vi "Progress Bar - Manager.vi"(6 "Steps to Increment (1)":dbl=1.0, 7 "Action (Init)":T1, 8 "error in (no error)":errorcluster, 9 "Number of Steps":dbl, 10 "Window Title (\"\")":string, 11 "Message":string) -> (0 "error out":errorcluster)   [LabVIEW 2014, in "Progress Bar.lvlib"]
uses:
  Progress Bar.lvlib
  _typedefs/PB_Manager Actions.ctl
  _typedefs/PB_Ref Cluster.ctl
panel:
  out "Init - Timed Out":bool
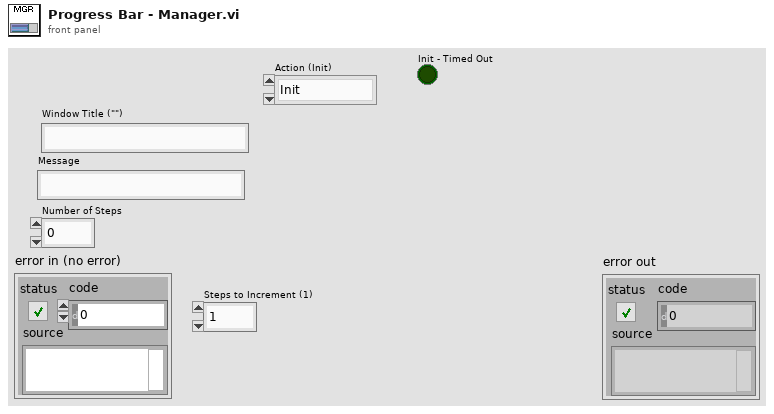
[diagram p1: front panel]
types:
  T1 = typedef "PB_Manager Actions.ctl" = enum16{"Init", "Update Bar", "Close"}
  T2 = typedef "PB_Ref Cluster.ctl" = cluster{"Message":refnum<user-event>, "ShutDown":refnum<user-event>, "User Abort":refnum<notifier>, "Load Complete":refnum<notifier>}
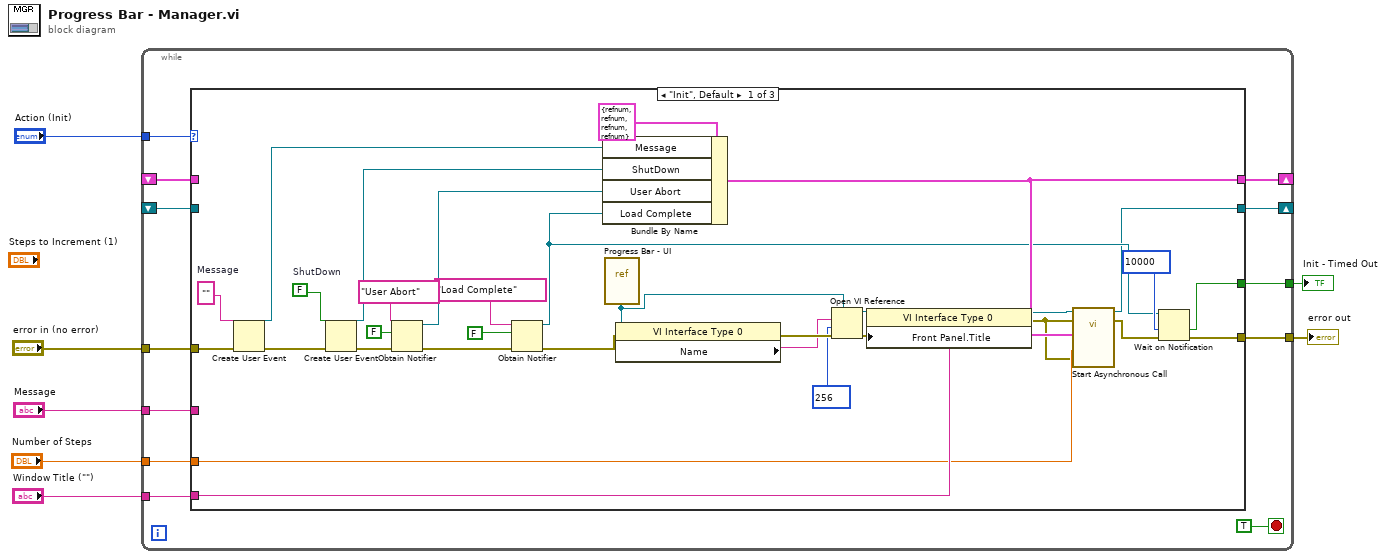
[diagram p0: block diagram]
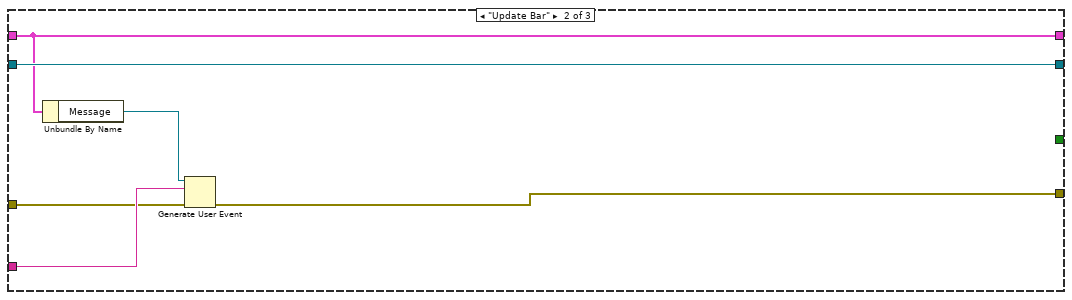
[diagram p2: hidden frame]
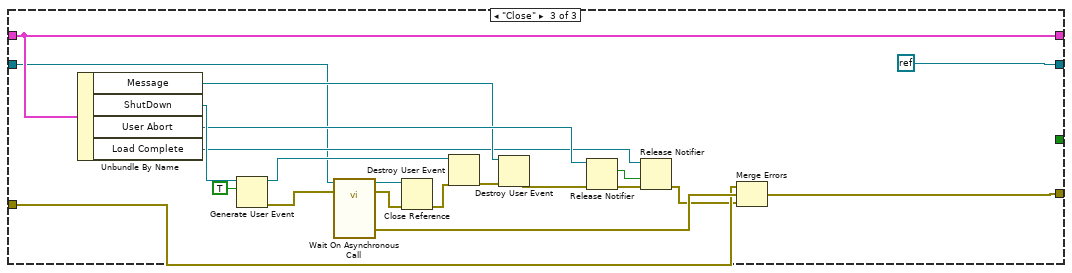
[diagram p3: hidden frame]
diagram:
  n1 = while {
    tunnel: "Action (Init)" -> [w19]
    shift-right: [w17] -> _
    shift-left: _ -> [w12]
    tunnel: "error in (no error)" -> [w16]
    tunnel: "Number of Steps" -> [w15]
    tunnel: [w14] -> w4
    shift-right: [w13] -> _
    shift-left: _ -> [w11]
    tunnel: "Message" -> [w10]
    tunnel: "Window Title (\"\")" -> [w9]
    tunnel: [w8] -> w1
    stop <- TRUE stop-if-true
    n2 = case shown="\"Init\", Default" w19 {
      tunnel: [w40 w52 w65] -> w17
      tunnel: w16 -> [w50 w54 w63]
      tunnel: w15 -> [w21 _ _]
      tunnel: [w29 w53 w66] -> w14
      tunnel: [w22 w57 refnum<k0> refnum] -> w13
      tunnel: w12 -> [_ w52 w65]
      tunnel: w11 -> [_ w57 w58]
      tunnel: w10 -> [_ w55 _]
      tunnel: w9 -> [w24 _ _]
      tunnel: [w28 _ _] -> w8
      frame "Init", Default {
        w48 = FALSE  # ShutDown
        w49 = ""  # Message
        n3 = Create User Event(user event datatype=w49, error in=w50) -> (user event=w41:refnum<user-event>, error out=w47:errorcluster)
        n4 = Create User Event(user event datatype=w48, error in=w47) -> (user event=w42:refnum<user-event>, error out=w45:errorcluster)
        n5 = Obtain Notifier(name (unnamed)="User Abort", notification data type=FALSE, error in (no error)=w45) -> (notifier out=w44:refnum<notifier>, error out=w33:errorcluster)  [unwired: 1 in, 1 out]
        n6 = Obtain Notifier(name (unnamed)="Load Complete", notification data type=FALSE, error in (no error)=w33) -> (notifier out=w30:refnum<notifier>, error out=w32:errorcluster)  [unwired: 1 in, 1 out]
        n7 = Bundle By Name(cluster=T2 {"Message"=refnum, "ShutDown"=refnum, "User Abort"=refnum, "Load Complete"=refnum} ("PB_Ref Cluster"), "Message"=w41, "ShutDown"=w42, "User Abort"=w44, "Load Complete"=w30) -> (w40:T2)
        n8 = vi-ref "Progress Bar - UI.vi"() -> (w37:refnum<vi>)
        n9 = property class="VI Interface Type 0"(reference=w37, error in=w32) -> (error out=w39:errorcluster, "Name"=w38:string)  [unwired: 1 out]
        n10 = Open VI Reference(type specifier VI Refnum (for type only)=w37, vi path=w38, options=256, error in (no error)=w39) -> (vi reference=w26:refnum<vi>, error out=w25:errorcluster)  [unwired: 2 in]
        n11 = property class="VI Interface Type 0"(reference=w26, error in=w25, "Front Panel.Title"=w24) -> (reference out=w23:refnum<vi>, error out=w20:errorcluster)
        n12 = call-by-ref "Start Asynchronous Call"(reference=w23, error in=w20, 8:"error in (no error)"=w20, "Number of Steps"=w21, "Ref Cluster"=w40) -> (reference out=w22:refnum<vi>, error out=w27:errorcluster)  [unwired: 8 in, 1 out]
        n13 = Wait on Notification(notifier=w30, timeout in ms (-1)=10000, error in (no error)=w27) -> (timed out?=w28:bool, error out=w29:errorcluster)  [unwired: 1 in, 2 out]
      }
      frame "Update Bar" {
        n14 = Unbundle By Name(w52) -> ("Message"=w56:refnum<user-event>)
        n15 = Generate User Event(user event=w56, event data cluster=w55, error in=w54) -> (error out=w53:errorcluster)  [unwired: 1 in, 1 out]
      }
      frame "Close" {
        n16 = Unbundle By Name(w65) -> ("Message"=w71:refnum<user-event>, "ShutDown"=w78:refnum<user-event>, "User Abort"=w72:refnum<notifier>, "Load Complete"=w60:refnum<notifier>)
        n17 = Generate User Event(user event=w78, event data cluster=TRUE ("event data")) -> (user event out=w73:refnum<user-event>, error out=w76:errorcluster)  [unwired: 2 in]
        n18 = call-by-ref "Wait On Asynchronous Call"(reference=w58, error in=w76) -> (reference out=w69:refnum<vi>, error out=w68:errorcluster, 0:"error out"=w75:errorcluster)  [unwired: 11 in]
        n19 = Close Reference(reference=w69, error in (no error)=w68) -> (error out=w67:errorcluster)
        n20 = Destroy User Event(user event=w73, error in=w67) -> (error out=w74:errorcluster)
        n21 = Destroy User Event(user event=w71, error in=w74) -> (error out=w70:errorcluster)
        n22 = Release Notifier(notifier=w72, error in (no error)=w70) -> (last notification=w62:bool, error out=w61:errorcluster)  [unwired: 1 in, 1 out]
        n23 = Release Notifier(notifier=w60, force destroy? (F)=w62, error in (no error)=w61) -> (error out=w59:errorcluster)  [unwired: 2 out]
        n24 = Merge Errors(w63, w75, w59) -> (w66:errorcluster)
      }
    }
  }
  "error out" <- w4
  "Init - Timed Out" <- w1
